vi "Add Help File to Example.vi"(8 "error in (no error)":errorcluster, 11 "Files Installed":path[](array[path])) -> (0 "error out":errorcluster)   [LabVIEW 2015]
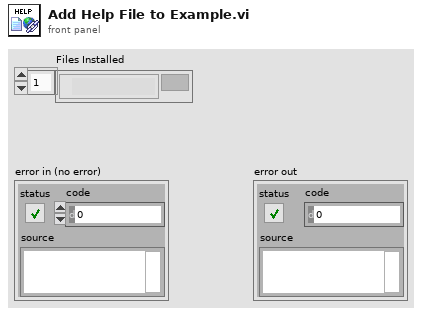
[diagram p1: front panel]
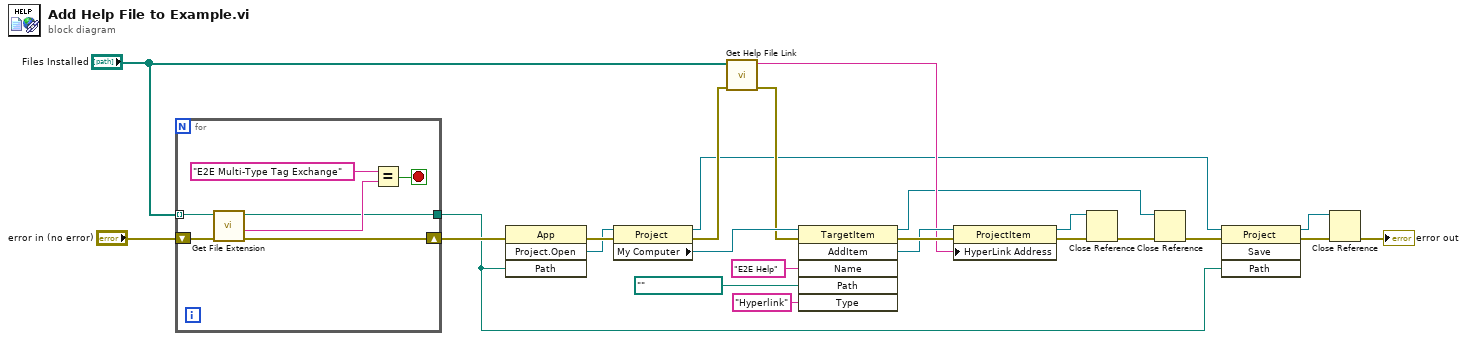
[diagram p0: block diagram]
diagram:
  n1 = for {
    tunnel: "Files Installed" -> [w31] mode=indexing
    shift-right: [w30] -> w23
    shift-left: "error in (no error)" -> [w29]
    tunnel: [w26] -> w1
    stop <- w25 stop-if-true
    n2 = call <vilib>:"Get File Extension.vi"("error in (no error)"=w29, "file"=w31) -> ("error out"=w30:errorcluster, "filename without extension"=w28:string, "dup file"=w26:path)  [unwired: 5 in, 2 out]
    n3 = Equal?(x="E2E Multi-Type Tag Exchange", y=w28) -> (x = y?=w25:bool)
  }
  n4 = invoke class="App" method="Project.Open"(error in=w23, "Path"=w1) -> (error out=w22:errorcluster, "Project:Open"=w21:refnum<vi>)  [unwired: 2 in, 2 out]
  n5 = property class="Project"(reference=w21, error in=w22) -> (reference out=w5:refnum<vi>, error out=w20:errorcluster, "My Computer"=w17:refnum<vi>)
  n6 = call "Get Help File Link.vi"("error in (no error)"=w20, "Files Installed"="Files Installed") -> ("error out"=w13:errorcluster, "Help File Link"=w14:string)  [unwired: 7 in, 1 out]
  n7 = invoke class="TargetItem" method="AddItem"(reference=w17, error in=w13, "Name"="E2E Help", "Path"=path "", "Type"="Hyperlink" ("Name")) -> (reference out=w6:refnum<vi>, error out=w16:errorcluster, "AddItem"=w15:refnum<vi>)  [unwired: 1 in, 3 out]
  n8 = property class="ProjectItem"(reference=w15, error in=w16, "HyperLink Address"=w14) -> (reference out=w8:refnum<vi>, error out=w10:errorcluster)
  n9 = Close Reference(reference=w8, error in (no error)=w10) -> (error out=w9:errorcluster)
  n10 = Close Reference(reference=w6, error in (no error)=w9) -> (error out=w7:errorcluster)
  n11 = invoke class="Project" method="Save"(reference=w5, error in=w7, "Path"=w1) -> (reference out=w3:refnum<vi>, error out=w4:errorcluster)  [unwired: 1 in, 2 out]
  n12 = Close Reference(reference=w3, error in (no error)=w4) -> (error out=→"error out":errorcluster)
